vi "pruebaun solo pin varia .vi"() -> ()   [LabVIEW 2013]
uses:
  <vilib>/LabVIEW Interface for Arduino/Type Defs/LCD Pin Config 4 bit.ctl
  <vilib>/LabVIEW Interface for Arduino/Type Defs/Arduino Resource.ctl
  <vilib>/LabVIEW Interface for Arduino/Type Defs/Board Type.ctl
  <vilib>/LabVIEW Interface for Arduino/Type Defs/Pin Mode.ctl
  <vilib>/LabVIEW Interface for Arduino/Type Defs/Direction.ctl
  <vilib>/Utility/file.llb/Write To Spreadsheet File (string).vi
  <vilib>/LabVIEW Interface for Arduino/LabVIEW Interface for Arduino.lvlib
panel:
  out "Arduino Resource 2":T1={"VISA resource"="", "Board Type"=enum."Uno", "Connection Type"=enum."USB / Serial", "Bytes Per Packet (15)"=15}
  out "error out 2":errorcluster
  out "error out":errorcluster
  out "Arduino Resource":T1
  in  "LCD Pin Config 4 Bit":T3={"RS"=12, "RW"=255, "Enable"=11, "D4"=5, "D5"=4, "D6"=3, "D7"=2, "LCD"=10}
  in  "stop":bool
  out "x*y":u8
  out "Voltage":dbl(knob) scale=0.0..5.0
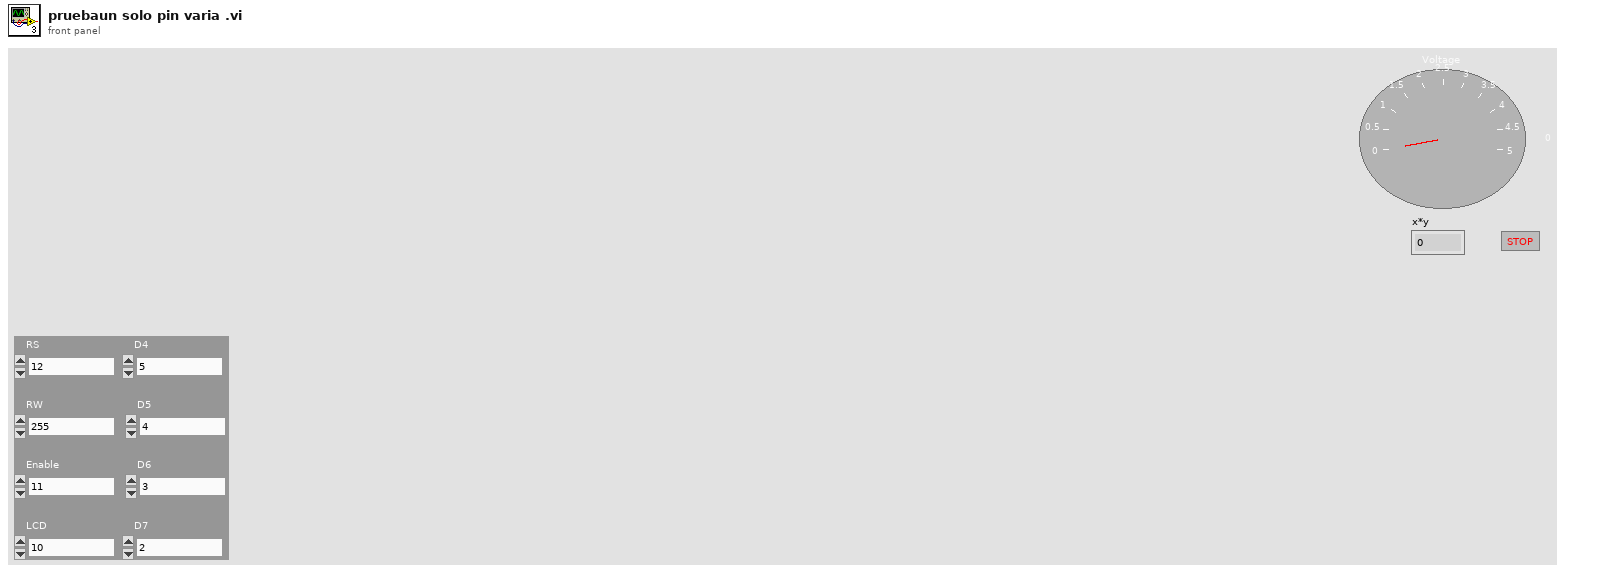
[diagram p1: front panel]
types:
  T1 = typedef "LabVIEW Interface for Arduino.lvlib/Arduino Resource.ctl" = cluster{"VISA resource":refnum<visa-resource-name>, "Board Type":T2, "Connection Type":enum8{"USB / Serial"}, "Bytes Per Packet (15)":u8}
  T2 = typedef "LabVIEW Interface for Arduino.lvlib/Board Type.ctl" = enum16{"Uno", "Dimuelanove w/Atmega 328", "Mega 2560"}
  T3 = typedef "LabVIEW Interface for Arduino.lvlib/LCD Pin Config 4 bit.ctl" = cluster{"RS":u8, "RW":u8, "Enable":u8, "D4":u8, "D5":u8, "D6":u8, "D7":u8, "LCD":u8}
  T4 = typedef "LabVIEW Interface for Arduino.lvlib/Pin Mode.ctl" = enum8{"Input", "Output"}
  T5 = typedef "LabVIEW Interface for Arduino.lvlib/Direction.ctl" = enum8{"Left ", "Right"}
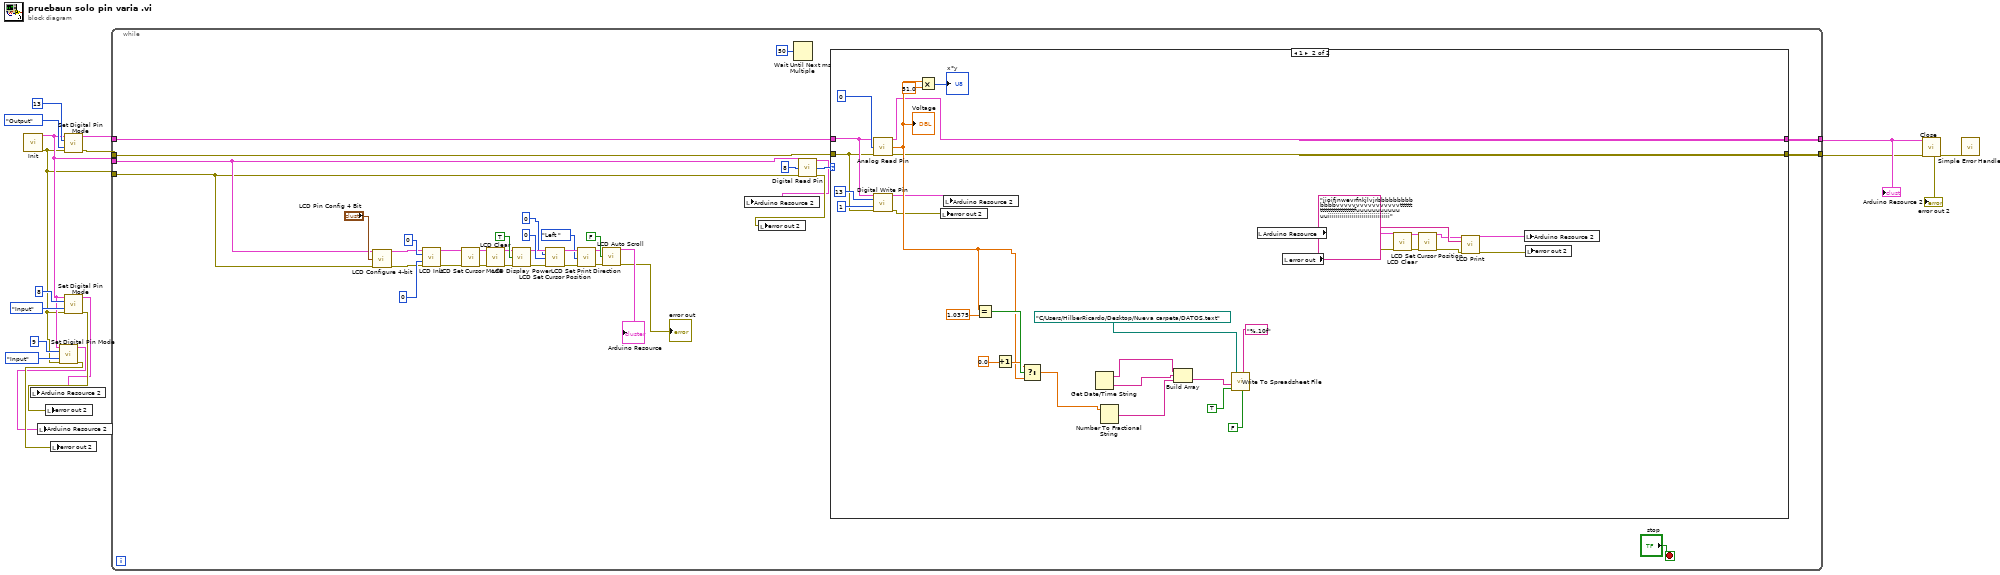
[diagram p0: block diagram]
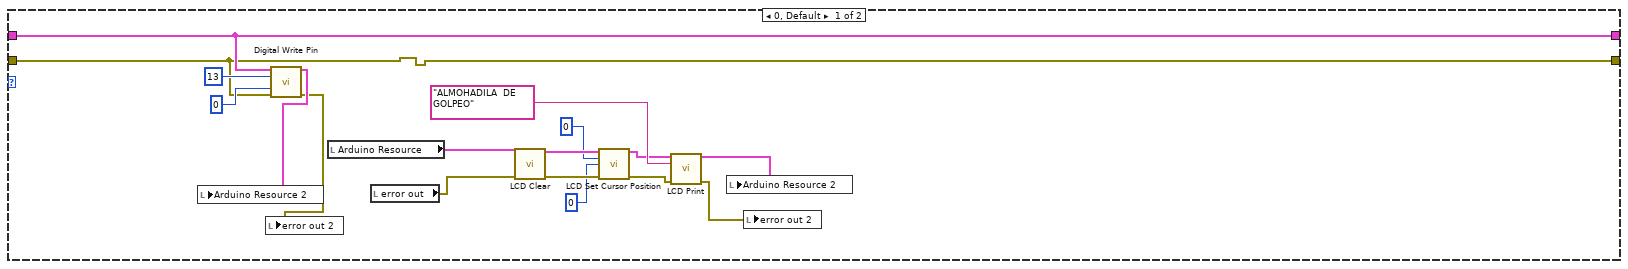
[diagram p2: hidden frame]
diagram:
  n1 = call <vilib>:"Init.vi"() -> ("Arduino Resource"=w6:T1, "error out"=w5:errorcluster)  [unwired: 18 in]
  n2 = call <vilib>:"Set Digital Pin Mode.vi"("Arduino Resource"=w6, "Digital I/O Pin"=u8 9, "Pin Mode (Input)"=Pin_Mode."Input", "error in"=w5) -> ("Arduino Resource"=w1:T1, "error out"=w3:errorcluster)  [unwired: 10 in]
  n3 = local write "Arduino Resource 2"(w1) -> ()
  n4 = local write "error out 2"(w3) -> ()
  n5 = call <vilib>:"Set Digital Pin Mode.vi"("Arduino Resource"=w6, "Digital I/O Pin"=u8 13, "Pin Mode (Input)"=Pin_Mode."Output", "error in"=w5) -> ("Arduino Resource"=w13:T1, "error out"=w12:errorcluster)  [unwired: 10 in]
  n6 = call <vilib>:"Set Digital Pin Mode.vi"("Arduino Resource"=w6, "Digital I/O Pin"=u8 8, "Pin Mode (Input)"=Pin_Mode."Input", "error in"=w5) -> ("Arduino Resource"=w2:T1, "error out"=w4:errorcluster)  [unwired: 10 in]
  n7 = local write "Arduino Resource 2"(w2) -> ()
  n8 = local write "error out 2"(w4) -> ()
  n9 = while {
    tunnel: w13 -> [w27]
    tunnel: w12 -> [w26]
    tunnel: [w53] -> w11
    tunnel: [w52] -> w10
    tunnel: w6 -> [w21]
    tunnel: w5 -> [w20]
    stop <- "stop" stop-if-true
    n10 = call <vilib>:"LCD Configure 4-bit.vi"("Arduino Resource"=w21, "LCD Pin Config 4 Bit"="LCD Pin Config 4 Bit", "error in"=w20) -> ("Arduino Resource"=w45:T1, "error out"=w44:errorcluster)  [unwired: 11 in]
    n11 = call <vilib>:"LCD Init.vi"("Arduino Resource"=w45, "Columns"=u8 0, "Rows"=u8 0, "error in"=w44) -> ("Arduino Resource"=w30:T1, "error out"=w29:errorcluster)  [unwired: 10 in]
    n12 = call <vilib>:"LCD Set Cursor Mode.vi"("Arduino Resource"=w30, "error out"=w29) -> ("Arduino Resource"=w36:T1, "error out"=w35:errorcluster)  [unwired: 12 in]
    n13 = call <vilib>:"LCD Clear.vi"("Arduino Resource"=w36, "error in"=w35) -> ("Arduino Resource"=w37:T1, "error out"=w38:errorcluster)  [unwired: 12 in]
    n14 = call <vilib>:"LCD Display Power.vi"("Arduino Resource"=w37, "Display On? (T) 2"=TRUE, "error in"=w38) -> ("Arduino Resource"=w40:T1, "error out"=w41:errorcluster)  [unwired: 11 in]
    n15 = call <vilib>:"LCD Set Cursor Position.vi"("Arduino Resource"=w40, "Column"=u8 0, "Row"=u8 0, "error out"=w41) -> ("Arduino Resource"=w33:T1, "error out"=w32:errorcluster)  [unwired: 10 in]
    n16 = call <vilib>:"LCD Set Print Direction.vi"("Arduino Resource"=w33, "Print Direction"=Direction."Left " ("Direction"), "error in"=w32) -> ("Arduino Resource"=w25:T1, "error"=w24:errorcluster)  [unwired: 11 in]
    n17 = call <vilib>:"LCD Auto Scroll.vi"("Arduino Resource"=w25, "Auto Scroll?"=FALSE ("Auto Scroll? 2"), "error in"=w24) -> ("Arduino Resource"=→"Arduino Resource":T1, "error out"=→"error out":errorcluster)  [unwired: 11 in]
    n18 = Wait Until Next ms Multiple(millisecond multiple=u32 50) -> ()  [unwired: 1 out]
    n19 = call <vilib>:"Digital Read Pin.vi"("Arduino Resource"=w21, "Digital I/O Pin (0)"=u8 8, "error in"=w20) -> ("Arduino Resource"=w18:T1, "Value"=w49:u8, "error out"=w19:errorcluster)  [unwired: 10 in]
    n20 = local write "Arduino Resource 2"(w18) -> ()
    n21 = local write "error out 2"(w19) -> ()
    n22 = case shown="1" w49 {
      tunnel: w26 -> [w58 w85]
      tunnel: w27 -> [w59 w86]
      tunnel: [w59 w72] -> w53
      tunnel: [w58 w71] -> w52
      frame 0, Default {
        n23 = call <vilib>:"Digital Write Pin.vi"("Arduino Resource"=w59, "Digital I/O Pin (0)"=u8 13, "Value (0)"=u8 0, "error in"=w58) -> ("Arduino Resource"=w55:T1, "error out"=w54:errorcluster)  [unwired: 10 in]
        n24 = local write "Arduino Resource 2"(w55) -> ()
        n25 = local write "error out 2"(w54) -> ()
        n26 = local read "Arduino Resource"() -> (w63:T1)
        n27 = local read "error out"() -> (w62:errorcluster)
        n28 = call <vilib>:"LCD Clear.vi"("Arduino Resource"=w63, "error in"=w62) -> ("Arduino Resource"=w64:T1, "error out"=w65:errorcluster)  [unwired: 12 in]
        n29 = call <vilib>:"LCD Set Cursor Position.vi"("Arduino Resource"=w64, "Column"=u8 0, "Row"=u8 0, "error out"=w65) -> ("Arduino Resource"=w66:T1, "error out"=w67:errorcluster)  [unwired: 10 in]
        n30 = call <vilib>:"LCD Print.vi"("Arduino Resource"=w66, "Data"="ALMOHADILA  DE GOLPEO", "error out"=w67) -> ("Arduino Resource"=w57:T1, "error out"=w56:errorcluster)  [unwired: 11 in]
        n31 = local write "Arduino Resource 2"(w57) -> ()
        n32 = local write "error out 2"(w56) -> ()
      }
      frame 1 {
        n33 = call <vilib>:"Analog Read Pin.vi"("Arduino Resource"=w86, "Analog Input Pin (0)"=u8 0, "error in"=w85) -> ("Arduino Resource"=w72:T1, "Voltage"=w84:dbl, "error out"=w71:errorcluster)  [unwired: 10 in]
        "Voltage" <- w84
        n34 = call <vilib>:"Digital Write Pin.vi"("Arduino Resource"=w86, "Digital I/O Pin (0)"=u8 13, "Value (0)"=u8 1, "error in"=w85) -> ("Arduino Resource"=w74:T1, "error out"=w73:errorcluster)  [unwired: 10 in]
        n35 = Multiply(x=w84, y=51.0) -> (x*y=→"x*y":u8)
        n36 = local write "error out 2"(w73) -> ()
        n37 = local write "Arduino Resource 2"(w74) -> ()
        n38 = Equal?(x=w84, y=1.0375) -> (x = y?=w90:bool)
        n39 = Increment(x=0.0) -> (x+1=w89:dbl)
        n40 = Select(t=w89, s=w90, f=w84) -> (s? t:f=w87:dbl)
        n41 = Get Date/Time String() -> (date string=w94:string, time string=w93:string)  [unwired: 3 in]
        n42 = Number To Fractional String(number=w87) -> (F-format string=w92:string)  [unwired: 3 in]
        n43 = Build Array(w94, w93, w92) -> (w97:string[])
        n44 = call-poly <vilib>:"Write To Spreadsheet File.vi"("transpose? (no:F)"=FALSE, "format (%s)"="%.10f" ("format (%.3f)"), "append to file? (new file:F)"=TRUE, "1D data"=w97, "file path (dialog if empty)"=path "C:/Users/HilberRicardo/Desktop/Nueva carpeta/DATOS.text") -> ()  [unwired: 3 in, 1 out]
        n45 = local read "Arduino Resource"() -> (w78:T1)
        n46 = local read "error out"() -> (w77:errorcluster)
        n47 = call <vilib>:"LCD Clear.vi"("Arduino Resource"=w78, "error in"=w77) -> ("Arduino Resource"=w79:T1, "error out"=w80:errorcluster)  [unwired: 12 in]
        n48 = call <vilib>:"LCD Set Cursor Position.vi"("Arduino Resource"=w79, "error out"=w80) -> ("Arduino Resource"=w81:T1, "error out"=w82:errorcluster)  [unwired: 12 in]
        n49 = call <vilib>:"LCD Print.vi"("Arduino Resource"=w81, "Data"="jioifjnwevrfnkjlvjrbbbbbbbbbbbbbvvvvvvvvvvvvvvvvtttttttttttttttttttttttfuuuuuuuuuuuuuiiiiiiiiiiiiiiiiiiiiiiiiiiiiiii", "error out"=w82) -> ("Arduino Resource"=w76:T1, "error out"=w75:errorcluster)  [unwired: 11 in]
        n50 = local write "Arduino Resource 2"(w76) -> ()
        n51 = local write "error out 2"(w75) -> ()
      }
    }
  }
  "error out 2" <- w10
  "Arduino Resource 2" <- w11
  n52 = call <vilib>:"Close.vi"("Arduino Resource"=w11, "error in"=w10) -> ("error out"=w9:errorcluster)  [unwired: 13 in]
  n53 = call <vilib>:"Simple Error Handler.vi"("error in (no error)"=w9) -> ()  [unwired: 4 in, 5 out]
